vi "Notifier-with-memory-3DnumArray.vi"(8 "error in":errorcluster, 10 "Timeout [ms]":i32, 11 "Notifier in":refnum<notifier>) -> (0 "error IO":errorcluster, 2 "Notification":sgl[][][](array[numeric]))   [LabVIEW 2013, in "CameraVision.lvlib" / "CV-UI.lvclass"]
doc: "Polymorphic type of Notifier-with-memory vi.\n\nAccepts a notifier reference for a 3-dimensional numeric array.\nThe vi listens for 'Timeout' miliseconds for a new message on the notifier.\nIf no message arrives or arrived before calling the vi, the last received message is returned.\n\nThe default message is an empty 3-dimensional array of singles."
uses:
  CV-UI.lvclass
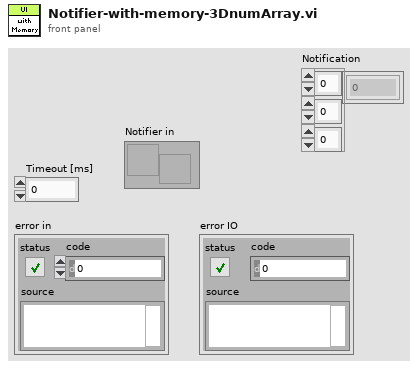
[diagram p1: front panel]
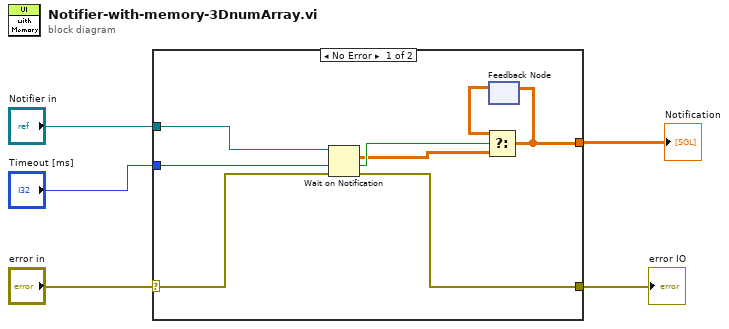
[diagram p0: block diagram]
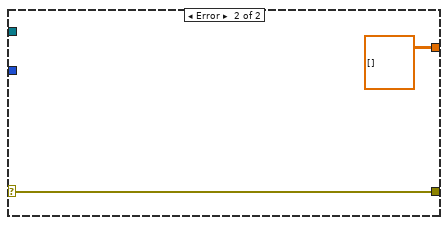
[diagram p2: hidden frame]
diagram:
  n1 = case shown="No Error" "error in" {
    selector: "error in" -> [w6 w14]
    tunnel: [w13 w14] -> w5
    tunnel: "Timeout [ms]" -> [w12 _]
    tunnel: [w9 sgl[][][] [] ("array")] -> w3
    tunnel: "Notifier in" -> [w8 _]
    frame No Error {
      n2 = Wait on Notification(notifier=w8, timeout in ms (-1)=w12, error in (no error)=w6) -> (notification=w10:sgl[][][], timed out?=w11:bool, error out=w13:errorcluster)  [unwired: 1 in, 1 out]
      n3 = feedback #1() -> (w7:sgl[][][])  [unwired: 1 in]
      n4 = Select(t=w7, s=w11, f=w10) -> (s? t:f=w9:sgl[][][])
      n5 = feedback-in #1(w9) -> ()
    }
    frame Error {
    }
  }
  "error IO" <- w5
  "Notification" <- w3
